vi "Logger.PGSQL.Read.vi"(8 "error in (no error)":errorcluster, 10 "address":string, 11 "Logger.PGSQL in":refnum<class "Logger.PGSQL.lvclass">) -> (0 "error out":errorcluster)   [LabVIEW 2019, in "Logger.PGSQL.lvlib" / "Logger.PGSQL.lvclass"]
uses:
  Logger.PGSQL.lvclass
  Logger.PGSQL.lvclass/Logger.PGSQL.ctl
  <userlib>/LevyLab/LV-Data/LV-Data.PG/API/Read Variable (string).vi
  <userlib>/LevyLab/LV-Data/LV-Data.PG/LV-Data.PGSQL.lvclass
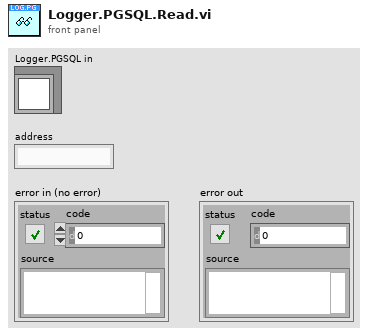
[diagram p1: front panel]
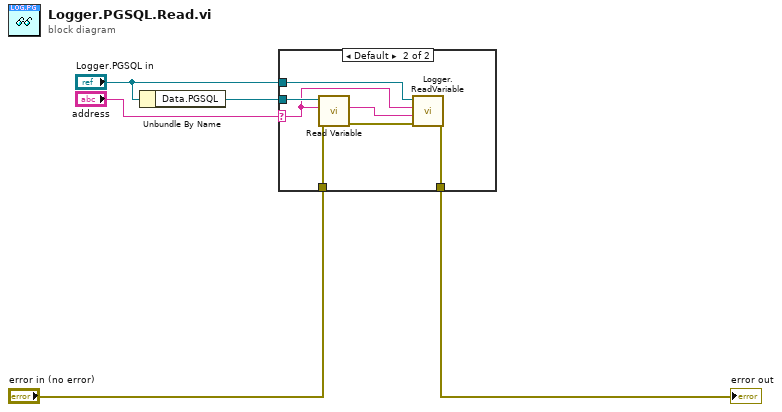
[diagram p0: block diagram]
diagram:
  n1 = Unbundle By Name("Logger.PGSQL in") -> ("Data.PGSQL"=w4:refnum<class "LV-Data.PGSQL.lvclass">)
  n2 = case shown="Default" "address" {
    selector: "address" -> [_ w7]
    tunnel: [w6 w13] -> w1
    tunnel: "Logger.PGSQL in" -> [_ w12]
    tunnel: w4 -> [_ w9]
    tunnel: "error in (no error)" -> [w6 w8]
    frame "" {
    }
    frame Default {
      n3 = call-poly <userlib>:"Read Variable.vi"("error in (no error)"=w8, "PG path"=w7, "Data.PGQL in"=w9) -> ("error out"=w10:errorcluster, "Value"=w11:string)  [unwired: 3 in, 4 out]
      n4 = call "Logger.ReadVariable.vi"("error in (no error)"=w10, "Data"=w11, "Address"=w7, "Logger"=w12) -> ("error out"=w13:errorcluster)  [unwired: 6 in, 1 out]
    }
  }
  "error out" <- w1
